vi "Engine - Copy & Script PPLTemplates (Inline-Async).vi"(7 "CD Name":string, 8 "error in (no error)":errorcluster, 9 "RT Driver VI Path":path, 10 "RT Driver Folder Path":path, 11 "CD Source Folder Path":path) -> (0 "error out":errorcluster)   [LabVIEW 2020, in "NIVS_Consolidated_CDW_MetaDataObj.lvclass"]
doc: "Via scripting, replace the tempate RTStateVariables control with the new type def across the async and RT driver VIs, and script the compiled settings property into the constants global"
uses:
  NIVS_Consolidated_CDW_MetaDataObj.lvclass
  Common.ctl
  <vilib>/Utility/traverseref.llb/TRef TravTarget.ctl
  CD Engine lvlib.ctl
  CD Shared lvlib.ctl
  Common.vi
  CD Engine lvlib.vi
  CD Shared lvlib.vi
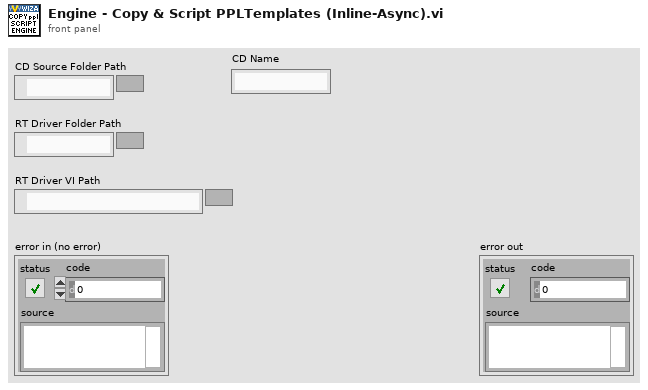
[diagram p1: front panel]
types:
  T1 = typedef "NIVS_Consolidated_CDW_MetaDataObj.lvclass/CD Engine lvlib.ctl" = enum16{"LibraryFileName", "LibraryFolderName", "Engine.FolderName", "Engine.Init.FolderName", "Engine.Run.FolderName", "Engine.Shutdown.FolderName", "Types.FolderName", "Engine.RT Driver VI.TemplatePath", "Engine.RT Driver VI.FileName", "Engine.PPL.RT Driver VI_InlineAsync.FileName", "Engine.RTStateVariables.Name", "Engine.PPL.RTStateVariables.Name", "Engine.RTStateVariables.Name.NoExtension", "Engine.Async.NameExtension", "Engine.Async.TemplateName", "Engine.PPL.Async.TemplateName", "Engine.PPL.Async.InitVSGlobals.Name", "Engine.PPL.RT Driver VI_Inline.FileName"}
  T2 = typedef "NIVS_Consolidated_CDW_MetaDataObj.lvclass/CD Shared lvlib.ctl" = enum16{"LibraryFileName", "LibraryFolderName", "ConstantsVI.VIPathAndName", "Shared.FolderName", "Shared.Types.FolderName", "Shared.Constants.VIName", "Shared.Constants.VITemplateName", "Shared.Constants.VITemplatePathAndName", "Shared.CompiledSettings.RelativePath", "Shared.Constants.RelativePath", "Shared.CompiledSettings.Name", "Shared.CompiledSettings.Name.NoExtension", "Shared.CompiledSettings.ClusterName"}
  T3 = typedef "TRef TravTarget.ctl" = enum16{"FP", "BD", "Other"}
  T4 = typedef "NIVS_Consolidated_CDW_MetaDataObj.lvclass/Common.ctl" = enum16{"ProjectName", "TemplatesFolderName", "PPLTemplatesFolderName", "ProjectTemplatePathAndName", "ProjectPPLTemplatePathAndName", "TimingAndSyncFolderName", "CustomDeviceFolderName", "PathToTemplates", "PathToPPLTemplates", "PathToExplorerPPLTemplates", "PathToEnginePPLTemplates", "PathToConfigurationFile", "ProjectConfigurationName"}
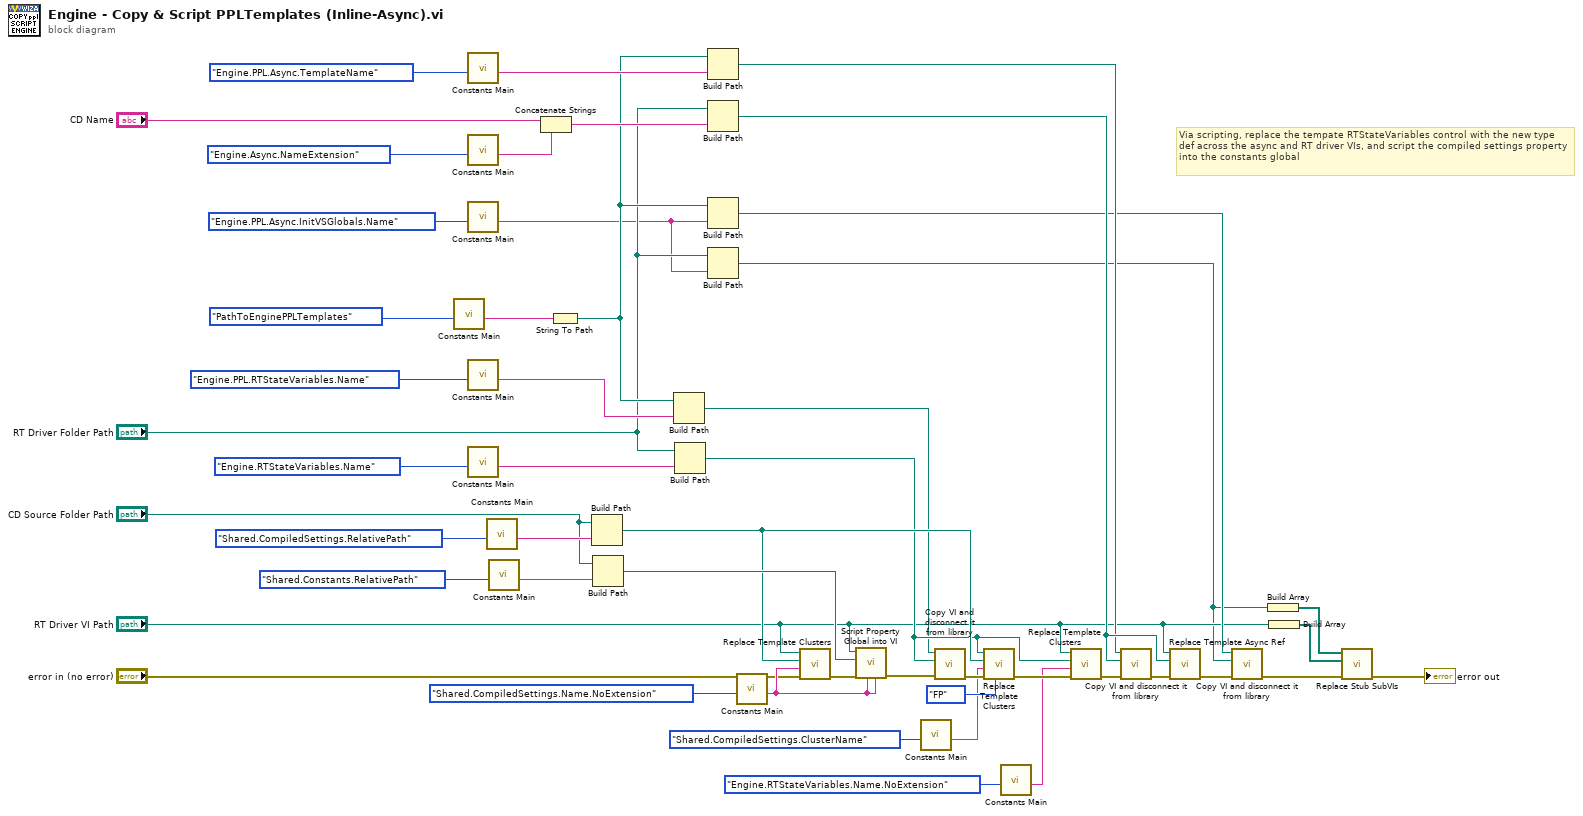
[diagram p0: block diagram]
diagram:
  # "Via scripting, replace the tempate RTStateVariables control with the new type def across the async and RT driver VIs, and script the compiled settings property into the constants global"
  n1 = call-poly "Constants Main.vi"("Action"=Common."PathToEnginePPLTemplates") -> ("Output"=w35:string)  [unwired: 10 in]
  n2 = call-poly "Constants Main.vi"("Action"=CD_Engine_lvlib."Engine.PPL.Async.TemplateName") -> ("Output"=w30:string)  [unwired: 10 in]
  n3 = call-poly "Constants Main.vi"("Action"=CD_Engine_lvlib."Engine.Async.NameExtension") -> ("Output"=w32:string)  [unwired: 10 in]
  n4 = call-poly "Constants Main.vi"("Action"=CD_Engine_lvlib."Engine.PPL.Async.InitVSGlobals.Name") -> ("Output"=w9:string)  [unwired: 10 in]
  n5 = call-poly "Constants Main.vi"("Action"=CD_Engine_lvlib."Engine.PPL.RTStateVariables.Name") -> ("Output"=w23:string)  [unwired: 10 in]
  n6 = call-poly "Constants Main.vi"("Action"=CD_Engine_lvlib."Engine.RTStateVariables.Name") -> ("Output"=w1:string)  [unwired: 10 in]
  n7 = call-poly "Constants Main.vi"("Action"=CD_Shared_lvlib."Shared.CompiledSettings.RelativePath") -> ("Output"=w28:string)  [unwired: 10 in]
  n8 = call-poly "Constants Main.vi"("Action"=CD_Shared_lvlib."Shared.Constants.RelativePath") -> ("Output"=w26:string)  [unwired: 10 in]
  n9 = Concatenate Strings("CD Name", w32) -> (w43:string)
  n10 = String To Path(string=w35) -> (path=w12:path)
  n11 = Build Path(base path="CD Source Folder Path", name or relative path=w28) -> (appended path=w48:path)
  n12 = Build Path(base path="CD Source Folder Path", name or relative path=w26) -> (appended path=w49:path)
  n13 = Build Path(base path=w12, name or relative path=w23) -> (appended path=w36:path)
  n14 = Build Path(base path="RT Driver Folder Path", name or relative path=w1) -> (appended path=w40:path)
  n15 = Build Path(base path=w12, name or relative path=w30) -> (appended path=w42:path)
  n16 = Build Path(base path="RT Driver Folder Path", name or relative path=w43) -> (appended path=w45:path)
  n17 = Build Path(base path=w12, name or relative path=w9) -> (appended path=w11:path)
  n18 = Build Path(base path="RT Driver Folder Path", name or relative path=w9) -> (appended path=w3:path)
  n19 = call-poly "Constants Main.vi"("Action"=CD_Shared_lvlib."Shared.CompiledSettings.Name.NoExtension") -> ("Output"=w21:string)  [unwired: 10 in]
  n20 = call "Replace Template Clusters.vi"("error in (no error)"="error in (no error)", "Control Name"=w21, "Path to Cluster to Replace"=w48, "Path to VI"="RT Driver VI Path") -> ("error out"=w46:errorcluster)  [unwired: 7 in]
  n21 = call "Script Property Global into VI.vi"("GlobalControlName"=w21, "StringConstantToReplace"=w21, "error in (no error)"=w46, "Path to Global"=w49, "Path to VI"="RT Driver VI Path") -> ("error out"=w47:errorcluster)  [unwired: 6 in]
  n22 = call-poly "Constants Main.vi"("Action"=CD_Shared_lvlib."Shared.CompiledSettings.ClusterName") -> ("Output"=w19:string)  [unwired: 10 in]
  n23 = call "Copy VI and disconnect it from library.vi"("error in (no error)"=w47, "VI Target Path"=w40, "VI Source Path"=w36) -> ("error out"=w37:errorcluster)  [unwired: 8 in]
  n24 = call "Replace Template Clusters.vi"("Traverse Target"=TRef_TravTarget."FP", "error in (no error)"=w37, "Control Name"=w19, "Path to Cluster to Replace"=w48, "Path to VI"=w40) -> ("error out"=w39:errorcluster)  [unwired: 6 in]
  n25 = call-poly "Constants Main.vi"("Action"=CD_Engine_lvlib."Engine.RTStateVariables.Name.NoExtension") -> ("Output"=w17:string)  [unwired: 10 in]
  n26 = call "Replace Template Clusters.vi"("error in (no error)"=w39, "Control Name"=w17, "Path to Cluster to Replace"=w40, "Path to VI"="RT Driver VI Path") -> ("error out"=w41:errorcluster)  [unwired: 7 in]
  n27 = call "Copy VI and disconnect it from library.vi"("error in (no error)"=w41, "VI Target Path"=w45, "VI Source Path"=w42) -> ("error out"=w44:errorcluster)  [unwired: 8 in]
  n28 = call "Replace Template Async Ref.vi"("error in (no error)"=w44, "Path to Desired Async VI"=w45, "Path to RT Driver VI"="RT Driver VI Path") -> ("error out"=w14:errorcluster)  [unwired: 8 in]
  n29 = call "Copy VI and disconnect it from library.vi"("error in (no error)"=w14, "VI Target Path"=w3, "VI Source Path"=w11) -> ("error out"=w8:errorcluster)  [unwired: 8 in]
  n30 = Build Array(w3) -> (w4:path[])
  n31 = Build Array("RT Driver VI Path") -> (w5:path[])
  n32 = call "Replace Stub SubVIs.vi"("error in"=w8, "VIs to Process"=w5, "subVIs to replace"=w4) -> ("error out"=→"error out":errorcluster)  [unwired: 8 in]
